vi "drawPixel.vi"(8 "y":i32, 9 "input_buffer":u8[](array[numeric]), 10 "color":bool, 11 "x":i32) -> (3 "output_buffer":u8[](array[numeric]) format="%b")   [LabVIEW 2017]
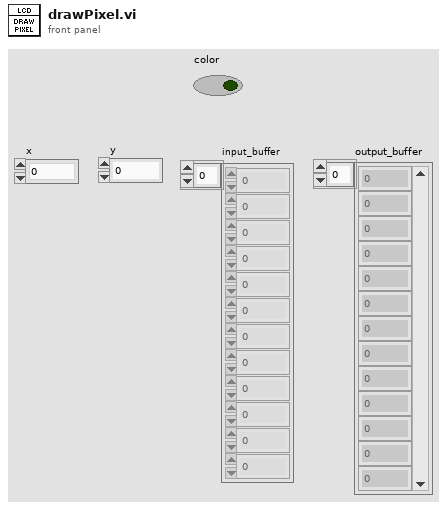
[diagram p1: front panel]
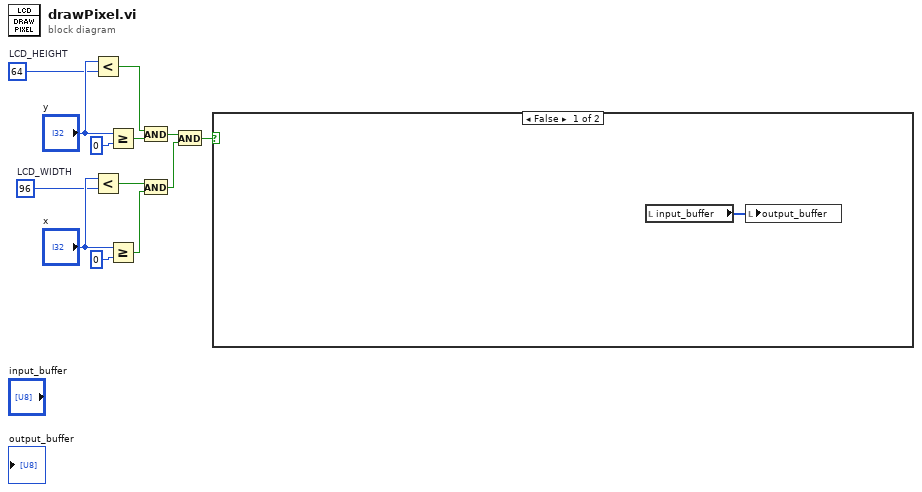
[diagram p0: block diagram]
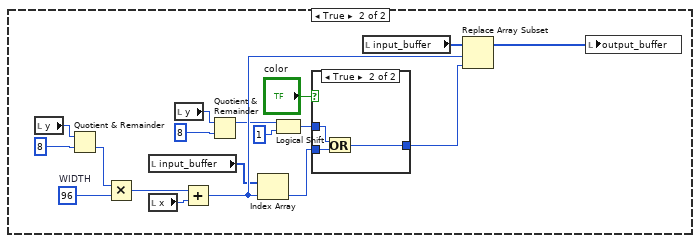
[diagram p2: hidden frame]
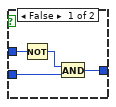
[diagram p3: hidden frame]
diagram:
  w11 = 64  # LCD_HEIGHT
  w6 = 96  # LCD_WIDTH
  n1 = Less?(x="y", y=w11) -> (x < y?=w10:bool)
  n2 = Less?(x="x", y=w6) -> (x < y?=w5:bool)
  n3 = Greater Or Equal?(x="y", y=0) -> (x >= y?=w9:bool)
  n4 = Greater Or Equal?(x="x", y=0) -> (x >= y?=w4:bool)
  n5 = And(x=w10, y=w9) -> (x .and. y?=w3:bool)
  n6 = And(x=w5, y=w4) -> (x .and. y?=w2:bool)
  n7 = And(x=w3, y=w2) -> (x .and. y?=w1:bool)
  n8 = case shown="False" w1 {
    frame False {
      n9 = local read "input_buffer"() -> (w14:u8[])
      n10 = local write "output_buffer"(w14) -> ()
    }
    frame True {
      w17 = 96  # WIDTH
      n11 = local read "y"() -> (w21:i32)
      n12 = Quotient & Remainder(x=w21, y=8) -> (floor(x/y)=w22:i32)  [unwired: 1 out]
      n13 = Multiply(x=w22, y=w17) -> (x*y=w23:i32)
      n14 = local read "input_buffer"() -> (w24:u8[])
      n15 = local read "x"() -> (w20:i32)
      n16 = local read "y"() -> (w25:i32)
      n17 = Add(x=w23, y=w20) -> (x+y=w27:i32)
      n18 = Quotient & Remainder(x=w25, y=8) -> (x-y*floor(x/y)=w26:i32)  [unwired: 1 out]
      n19 = Index Array "Index Array"(array=w24, index=w27) -> (element=w31:u8)
      n20 = Logical Shift(y=w26, x=u8 1) -> (x << y=w30:u8)
      n21 = case shown="True" "color" {
        tunnel: w30 -> [w36 w39]
        tunnel: w31 -> [w34 w38]
        tunnel: [w33 w37] -> w32
        frame False {
          n22 = Not(x=w36) -> (.not. x?=w35:u8)
          n23 = And(x=w35, y=w34) -> (x .and. y?=w33:u8)
        }
        frame True {
          n24 = Or(x=w39, y=w38) -> (x .or. y?=w37:u8)
        }
      }
      n25 = local read "input_buffer"() -> (w28:u8[])
      n26 = Replace Array Subset "Replace Array Subset"(array=w28, new element=w32, index=w27) -> (w15:u8[])
      n27 = local write "output_buffer"(w15) -> ()
    }
  }
